vi "User Event-Panel Resize.vi"(8 "Error In":errorcluster, 10 "Panel Resize Data":T1={"OldBnds"={"Left"=0, "Top"=0, "Right"=0, "Bottom"=0}, "NewBnds"={"Left"=0, "Top"=0, "Right"=0, "Bottom"=0}, "Act"=enum."Resized", "PrevState"=enum."Standard"}, 11 "Appearance Actor in":refnum<class "Appearance Actor.lvclass">) -> (0 "Error Out":errorcluster, 3 "Appearance Actor out":refnum<class "Appearance Actor.lvclass">)   [LabVIEW 2021, in "Appearance Actor.lvlib" / "Appearance Actor.lvclass"]
uses:
  Appearance Actor.lvclass
  C:/Program Files (x86)/National Instruments/LabVIEW 2021/vi.lib/ActorFramework/Actor/Actor.lvclass
  Typedefs/User Event-Panel Resize-Data--cluster.ctl
  <vilib>/Utility/miscctls.llb/LVRectTypeDef.ctl
  <vilib>/event_ctls.llb/sizeaction.ctl
  <vilib>/event_ctls.llb/panelstate.ctl
  <vilib>/ActorFramework/Actor/Actor.lvclass/Actor.ctl
  <vilib>/ActorFramework/Message Enqueuer/Message Enqueuer.lvclass/Message Enqueuer.ctl
  Appearance Actor Messages/UI-Set Maximize Button Value Msg/UI-Set Maximize Button Value Msg.lvclass/UI-Set Maximize Button Value Msg.ctl
  <vilib>/ActorFramework/Message Enqueuer/Init from Existing Queue.vi
  <vilib>/ActorFramework/Message Enqueuer/Enqueue.vi
  Appearance Actor Messages/UI-Set Maximize Button Value Msg/UI-Set Maximize Button Value Msg.lvclass
  C:/Program Files (x86)/National Instruments/LabVIEW 2021/vi.lib/ActorFramework/Message/Message.lvclass
  <vilib>/ActorFramework/Message Priority Queue/Priority Enqueue.vi
  <vilib>/ActorFramework/Message Enqueuer/Message Enqueuer.lvclass
  <vilib>/ActorFramework/Actor/Actor.lvclass
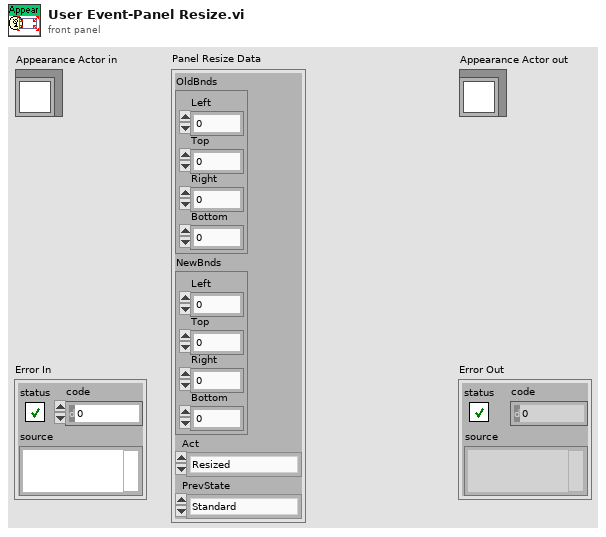
[diagram p1: front panel]
types:
  T1 = typedef "Appearance Actor.lvlib/Appearance Actor.lvclass/User Event-Panel Resize-Data--cluster.ctl" = cluster{"OldBnds":T2, "NewBnds":T2, "Act":T3, "PrevState":T4}
  T2 = typedef "LVRectTypeDef.ctl" = cluster{"Left":i16, "Top":i16, "Right":i16, "Bottom":i16}
  T3 = typedef "sizeaction.ctl" = enum32{"Minimized", "Maximized", "Resized"}
  T4 = typedef "panelstate.ctl" = enum32{"Standard", "Minimized", "Maximized"}
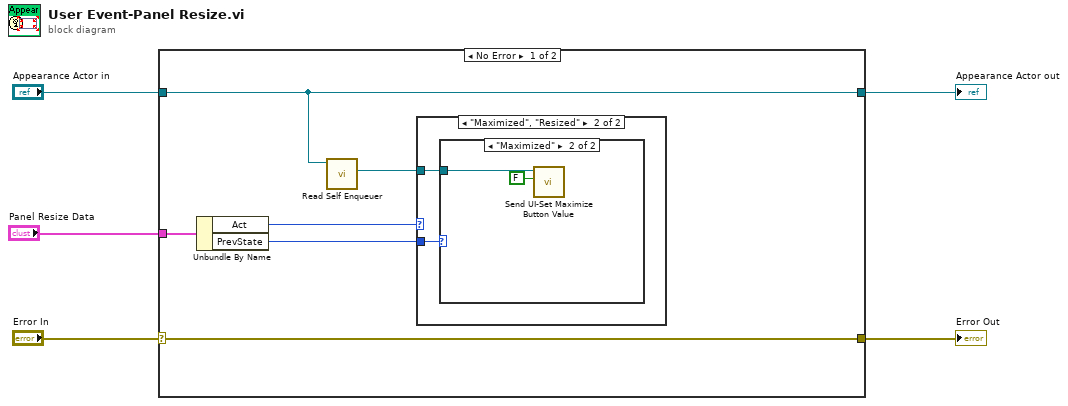
[diagram p0: block diagram]
diagram:
  n1 = case shown="No Error" "Error In" {
    selector: "Error In" -> [w11 w17]
    tunnel: [w11 w17] -> w4
    tunnel: "Appearance Actor in" -> [w9 w16]
    tunnel: [w9 w16] -> w2
    tunnel: "Panel Resize Data" -> [w10 _]
    frame No Error {
      n2 = Unbundle By Name(w10) -> ("Act"=w8:T3, "PrevState"=w6:T4)
      n3 = call <vilib>:"Read Self Enqueuer.vi"("Actor"=w9) -> ("Self Enqueuer"=w7:refnum<class "Message Enqueuer.lvclass">)  [unwired: 10 in]
      n4 = case shown="\"Maximized\", \"Resized\"" w8 {
        tunnel: w7 -> [_ w12]
        tunnel: w6 -> [_ w13]
        frame Default {
        }
        frame "Maximized", "Resized" {
          n5 = case shown="\"Maximized\"" w13 {
            tunnel: w12 -> [_ w15]
            frame Default {
            }
            frame "Maximized" {
              n6 = call "Send UI-Set Maximize Button Value.vi"("Value (F)"=FALSE, "Message Enqueuer"=w15) -> ()  [unwired: 8 in, 2 out]
            }
          }
        }
      }
    }
    frame Error {
    }
  }
  "Error Out" <- w4
  "Appearance Actor out" <- w2
